vi "GetSingleControlReferenceType.vi"(8 "error in (no error)":errorcluster, 10 "ID":string, 11 "ByteGSWebAPI-V0 in":refnum<class "ByteGSWebAPI-V0.lvclass">) -> (0 "error out":errorcluster, 2 "SingleControlReferenceType":T1, 3 "ByteGSWebAPI-V0 out":refnum<class "ByteGSWebAPI-V0.lvclass">)   [LabVIEW 2019, in "ByteGSWebAPI.lvlib" / "ByteGSWebAPI-V0.lvclass"]
doc: "Richiesta di GET control reference identificato da un ID in ingresso"
uses:
  ByteGSWebAPI-V0.lvclass
  Cntrls/SingleControlReferenceType.ctl
  54c15d21-1fd3-4ea8-80e2-c69b0da6434b.vi
  <vilib>/JDP Science/JSONtext/JSON text to Variant.vi
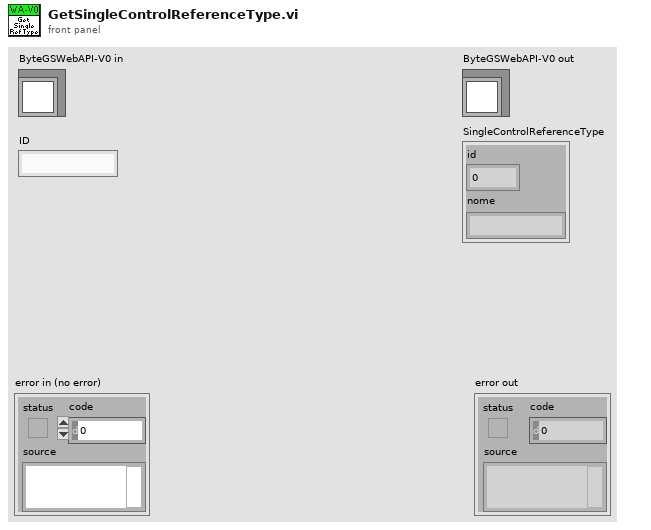
[diagram p1: front panel]
types:
  T1 = typedef "ByteGSWebAPI.lvlib/ByteGSWebAPI-V0.lvclass/SingleControlReferenceType.ctl" = cluster{"id":i32, "nome":string}
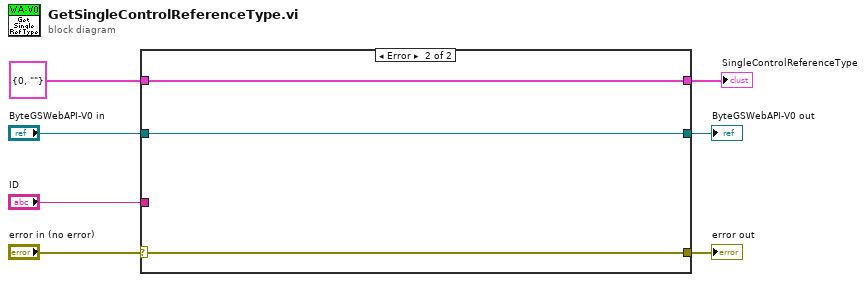
[diagram p0: block diagram]
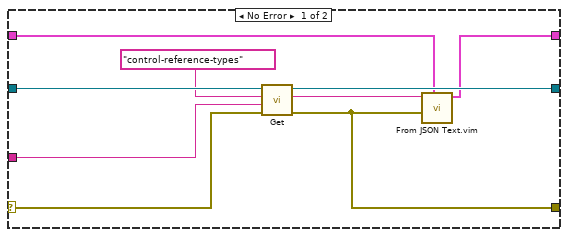
[diagram p2: hidden frame]
diagram:
  n1 = case shown="Error" "error in (no error)" {
    selector: "error in (no error)" -> [w13 w19]
    tunnel: [w8 w19] -> w6
    tunnel: [w15 w18] -> w4
    tunnel: "ByteGSWebAPI-V0 in" -> [w16 w18]
    tunnel: "ID" -> [w12 _]
    tunnel: T1 {"id"=0, "nome"=""} ("SingleControlReferenceType") -> [w10 w17]
    tunnel: [w9 w17] -> w1
    frame No Error {
      n2 = call "Get.vi"("error in (no error)"=w13, "Parameter"=w12, "Request"="control-reference-types" ("Parameter"), "ByteGSWebAPI-V0 in"=w16) -> ("error out"=w8:errorcluster, "body"=w11:string, "ByteGSWebAPI-V0 out"=w15:refnum<class "ByteGSWebAPI-V0.lvclass">)  [unwired: 4 in, 1 out]
      n3 = call "From JSON Text.vim"("Data Type and Default Value"=w10, "error in (no error)"=w8, "JSON"=w11) -> ("Data out"=w9:T1)  [unwired: 7 in, 1 out]
    }
    frame Error {
    }
  }
  "error out" <- w6
  "ByteGSWebAPI-V0 out" <- w4
  "SingleControlReferenceType" <- w1
